vi "Plan Path.vi"(8 "error in (no error)":errorcluster, 10 "Controle":T1, 11 "map reference in":refnum<data-value>) -> (0 "error out":errorcluster, 1 "intensity values":dbl[][](array[numeric]), 2 "Indicator":T1, 3 "map reference out":refnum<data-value>)   [LabVIEW 2012]
uses:
  <vilib>/robotics/Navigation/shared/WorldMap/OccupancyGridWorldMap/NI_Robotics_OccupancyGridWorldMap.lvclass
  <vilib>/robotics/Navigation/NI_Robotics_Navigation .lvlib
panel:
  out "x-y":dbl[][](array[numeric])
  out "goal node":cluster{"X":i32, "Y":i32}={"X"=32, "Y"=32}
  out "start node":cluster{"X":i32, "Y":i32}={"X"=3, "Y"=3}
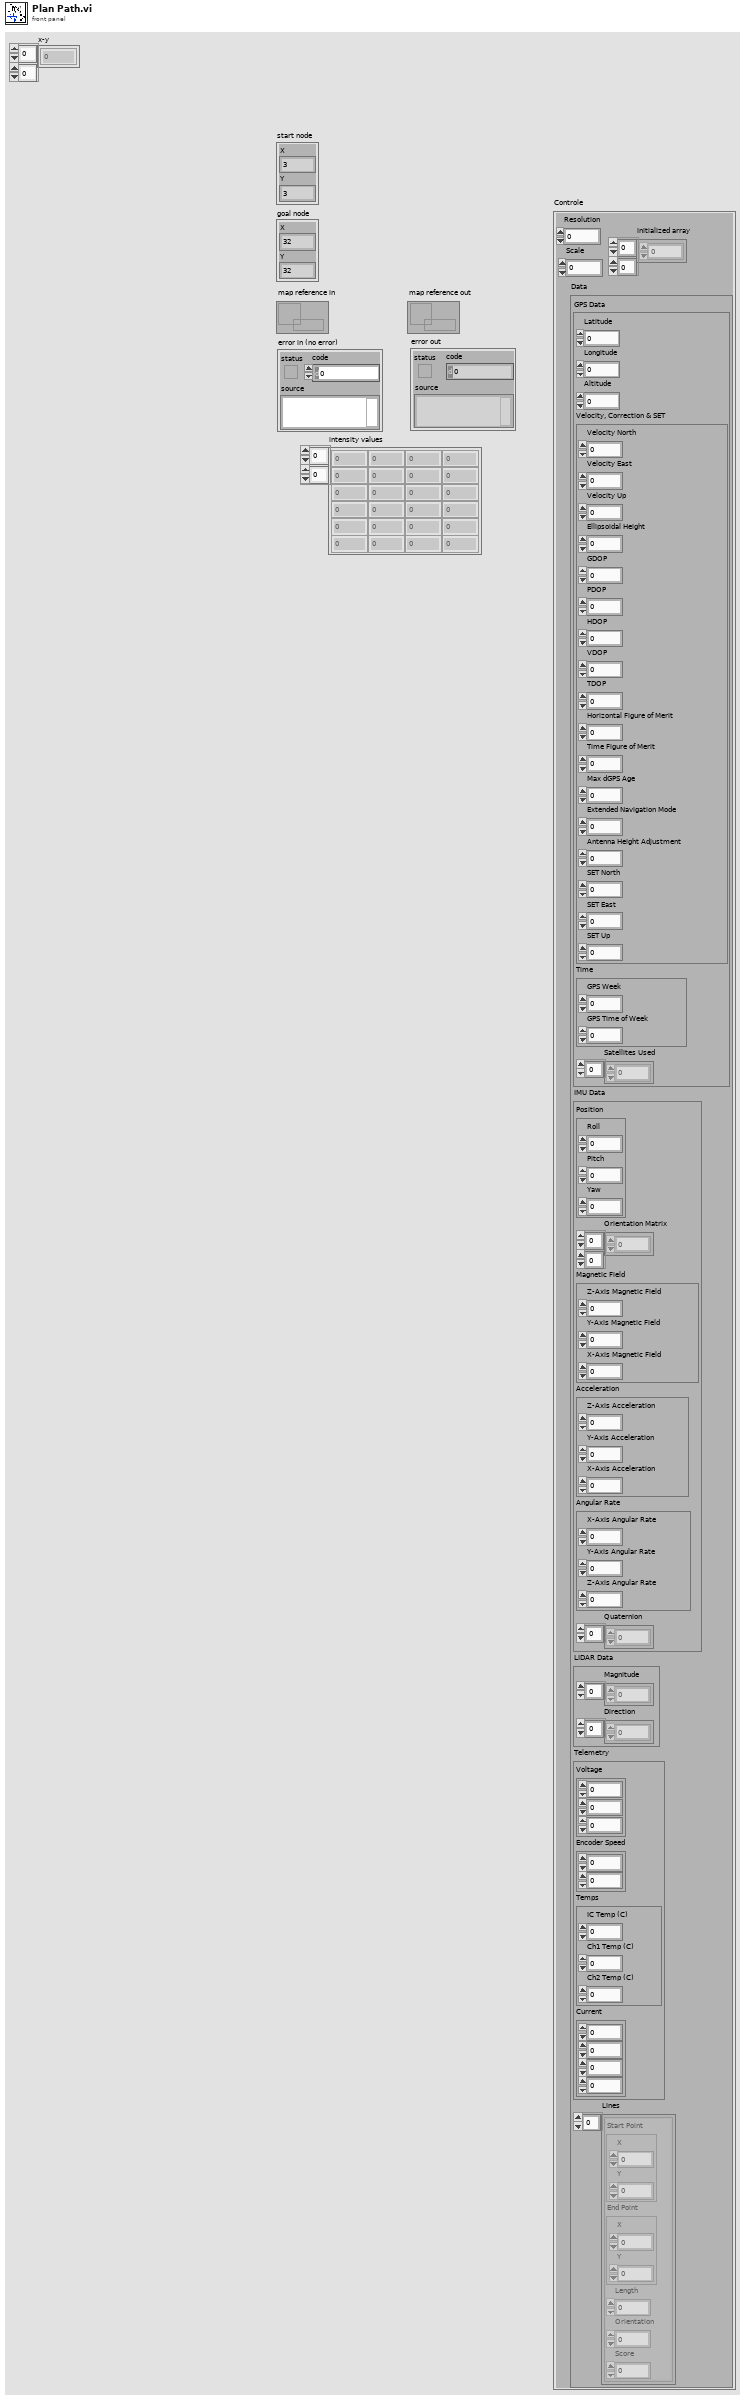
[diagram p1: front panel]
types:
  T1 = cluster{"Resolution":i32, "Scale":dbl, "Data":cluster{"GPS Data":cluster{"Latitude":dbl, "Longitude":dbl, "Altitude":dbl, "Velocity, Correction & SET":cluster{"Velocity North":dbl, "Velocity East":dbl, "Velocity Up":dbl, "Ellipsoidal Height":dbl, "GDOP":sgl, "PDOP":sgl, "HDOP":sgl, "VDOP":sgl, "TDOP":sgl, "Horizontal Figure of Merit":u8, "Time Figure of Merit":u8, "Max dGPS Age":sgl, "Extended Navigation Mode":u8, "Antenna Height Adjustment ":dbl, "SET North":i32, "SET East":i32, "SET Up":i32}, "Time":cluster{"GPS Week":u16, "GPS Time of Week":sgl}, "Satellites Used":i32[]}, "IMU Data":cluster{"Position":cluster{"Roll":dbl, "Pitch":dbl, "Yaw":dbl}, "Orientation Matrix":dbl[][], "Magnetic Field":cluster{"Z-Axis Magnetic Field":dbl, "Y-Axis Magnetic Field":dbl, "X-Axis Magnetic Field":dbl}, "Acceleration":cluster{"Z-Axis Acceleration":dbl, "Y-Axis Acceleration":dbl, "X-Axis Acceleration":dbl}, "Angular Rate":cluster{"X-Axis Angular Rate":dbl, "Y-Axis Angular Rate":dbl, "Z-Axis Angular Rate":dbl}, "Quaternion":dbl[]}, "LIDAR Data":cluster{"Magnitude":dbl[], "Direction":dbl[]}, "Telemetry":cluster{"Voltage":cluster{sgl, sgl, sgl}, "Encoder Speed":cluster{i32, i32}, "Temps":cluster{"IC Temp (C)":i32, "Ch1 Temp (C)":i32, "Ch2 Temp (C)":i32}, "Current":cluster{dbl, dbl, dbl, dbl}}, "Lines":cluster{"Start Point":cluster{"X":sgl, "Y":sgl}, "End Point":cluster{"X":sgl, "Y":sgl}, "Length":dbl, "Orientation":dbl, "Score":dbl}[]}, "initialized array":dbl[][]}
  T2 = cluster{"Latitude":dbl, "Longitude":dbl, "Altitude":dbl, "Velocity, Correction & SET":cluster{"Velocity North":dbl, "Velocity East":dbl, "Velocity Up":dbl, "Ellipsoidal Height":dbl, "GDOP":sgl, "PDOP":sgl, "HDOP":sgl, "VDOP":sgl, "TDOP":sgl, "Horizontal Figure of Merit":u8, "Time Figure of Merit":u8, "Max dGPS Age":sgl, "Extended Navigation Mode":u8, "Antenna Height Adjustment ":dbl, "SET North":i32, "SET East":i32, "SET Up":i32}, "Time":cluster{"GPS Week":u16, "GPS Time of Week":sgl}, "Satellites Used":i32[]}
  T3 = cluster{"Position":cluster{"Roll":dbl, "Pitch":dbl, "Yaw":dbl}, "Orientation Matrix":dbl[][], "Magnetic Field":cluster{"Z-Axis Magnetic Field":dbl, "Y-Axis Magnetic Field":dbl, "X-Axis Magnetic Field":dbl}, "Acceleration":cluster{"Z-Axis Acceleration":dbl, "Y-Axis Acceleration":dbl, "X-Axis Acceleration":dbl}, "Angular Rate":cluster{"X-Axis Angular Rate":dbl, "Y-Axis Angular Rate":dbl, "Z-Axis Angular Rate":dbl}, "Quaternion":dbl[]}
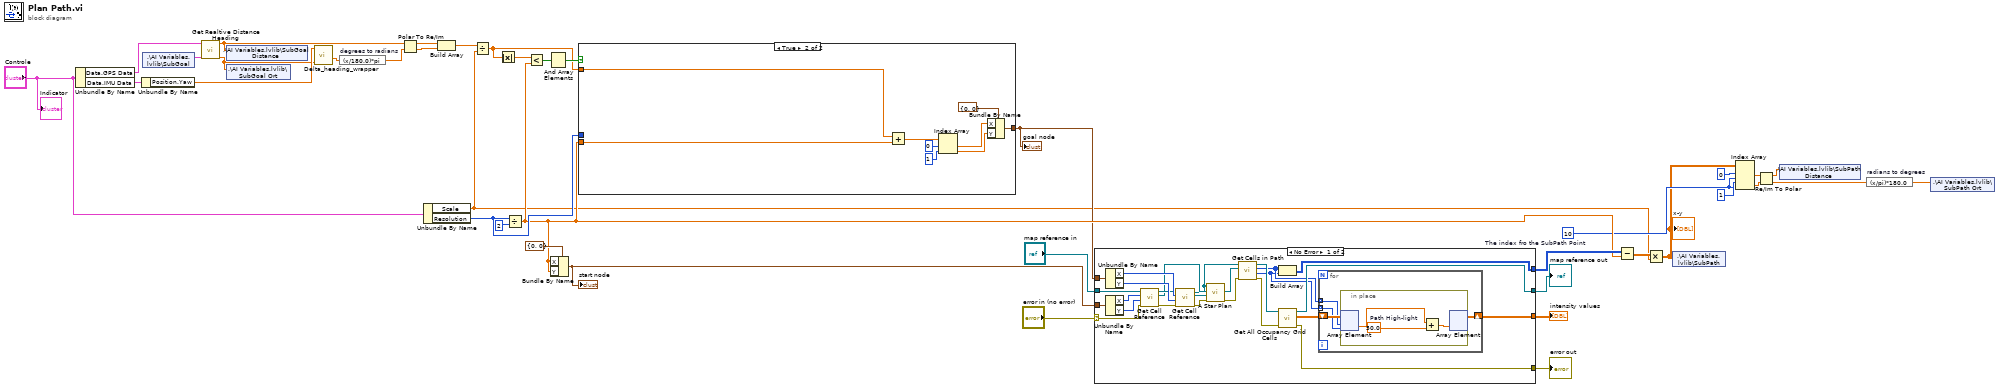
[diagram p0: block diagram]
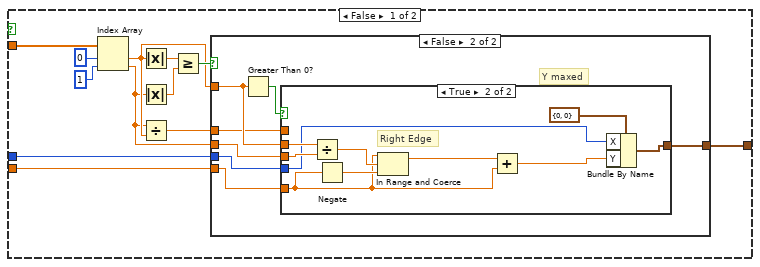
[diagram p2: hidden frame]
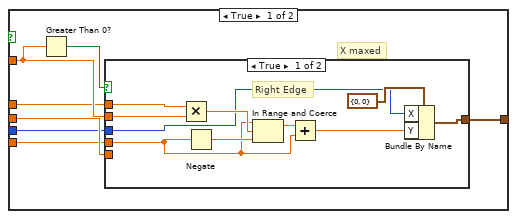
[diagram p3: hidden frame]
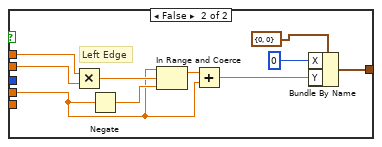
[diagram p4: hidden frame]
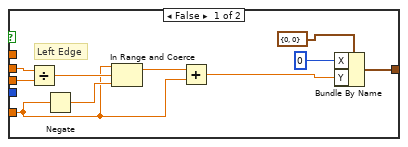
[diagram p5: hidden frame]
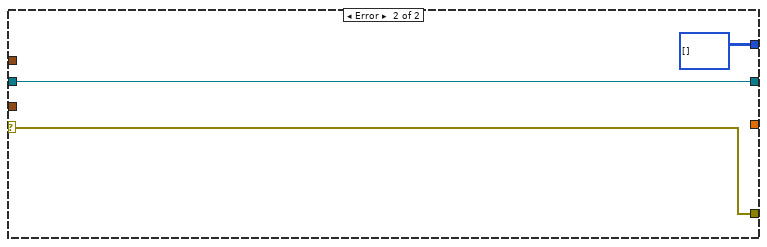
[diagram p6: hidden frame]
diagram:
  w9 = 10  # The index fro the SubPath Point
  n1 = Unbundle By Name("Controle") -> ("Data.GPS Data"=w12:T2, "Data.IMU Data"=w15:T3)
  n2 = Unbundle By Name(w15) -> ("Position.Yaw"=w11:dbl)
  n3 = shared-variable ".\\AI Variables.lvlib\\SubGoal"() -> (w13:T2)  [unwired: 1 in, 1 out]
  n4 = call "Get Realtive Distance Heading.vi"("Goal Position"=w13, "Current Position"=w12) -> ("Bearing"=w1:dbl, "distance (m)"=w5:dbl)  [unwired: 8 in]
  n5 = shared-variable ".\\AI Variables.lvlib\\SubGoal Distance"(w5) -> ()  [unwired: 1 in, 1 out]
  n6 = shared-variable ".\\AI Variables.lvlib\\SubGoal Ort"(w1) -> ()  [unwired: 1 in, 1 out]
  n7 = call "Delta_heading_wrapper.vi"("Goal Heading"=w1, "Robot Heading"=w11) -> ("Heading Adjustment"=w10:dbl)  [unwired: 9 in]
  n8 = expression code="(x/180.0)*pi" "degrees to radians"(w10) -> (w18:dbl)
  n9 = Polar To Re/Im(2:w18, 3:w5) -> (0:w16:dbl, 1:w17:dbl)
  n10 = Unbundle By Name("Controle") -> ("Scale"=w2:dbl, "Resolution"=w22:i32)
  n11 = Build Array(w17, w16) -> (w21:dbl[])
  n12 = Divide(x=w21, y=w2) -> (x/y=w23:dbl[])
  n13 = Absolute Value(x=w23) -> (abs(x)=w24:dbl[])
  n14 = Divide(x=w22, y=2 ("value")) -> (x/y=w20:dbl)
  n15 = Less?(x=w24, y=w20) -> (x < y?=w33:bool[])
  n16 = And Array Elements(Boolean array=w33) -> (logical AND=w34:bool)
  n17 = Bundle By Name(cluster=cluster{"X":i32, "Y":i32} {"X"=0, "Y"=0} ("goal node"), "X"=w20, "Y"=w20) -> (w31:cluster{"X":i32, "Y":i32})
  "start node" <- w31
  n18 = case shown="True" w34 {
    tunnel: w23 -> [w42 w114]
    tunnel: [w43 w107] -> w19
    tunnel: w22 -> [w41 _]
    tunnel: w20 -> [w40 w106]
    frame False {
      n19 = Index Array(array=w42, index #1=0 ("index"), index #2=1 ("index")) -> (element #1=w46:dbl, element #2=w45:dbl)
      n20 = Absolute Value(x=w46) -> (abs(x)=w49:dbl)
      n21 = Absolute Value(x=w45) -> (abs(x)=w48:dbl)
      n22 = Divide(x=w45, y=w46) -> (x/y=w44:dbl)
      n23 = Greater Or Equal?(x=w49, y=w48) -> (x >= y?=w47:bool)
      n24 = case shown="False" w47 {
        tunnel: w46 -> [w56 w83]
        tunnel: w45 -> [w55 w82]
        tunnel: w44 -> [w54 w81]
        tunnel: [w57 w84] -> w43
        tunnel: w41 -> [w53 w80]
        tunnel: w40 -> [w52 w79]
        frame True {
          # "X maxed"
          n25 = Greater Than 0?(x=w56) -> (x > 0?=w58:bool)
          n26 = case shown="True" w58 {
            tunnel: [w67 w77] -> w57
            tunnel: w56 -> [w65 w75]
            tunnel: w55 -> [_ _]
            tunnel: w54 -> [w66 w76]
            tunnel: w53 -> [w62 _]
            tunnel: w52 -> [w59 w70]
            frame True {
              # "Right Edge"
              n27 = Multiply(x=w66, y=w65) -> (x*y=w64:dbl)
              n28 = Negate(x=w59) -> (-x=w60:dbl)
              n29 = In Range and Coerce(upper limit=w59, x=w64, lower limit=w60) -> (coerced(x)=w63:dbl)  [unwired: 1 out]
              n30 = Add(x=w63, y=w59) -> (x+y=w61:dbl)
              n31 = Bundle By Name(cluster=cluster{"X":i32, "Y":i32} {"X"=0, "Y"=0} ("goal node"), "X"=w62, "Y"=w61) -> (w67:cluster{"X":i32, "Y":i32})
            }
            frame False {
              # "Left Edge"
              n32 = Multiply(x=w76, y=w75) -> (x*y=w74:dbl)
              n33 = Negate(x=w70) -> (-x=w71:dbl)
              n34 = In Range and Coerce(upper limit=w70, x=w74, lower limit=w71) -> (coerced(x)=w73:dbl)  [unwired: 1 out]
              n35 = Add(x=w73, y=w70) -> (x+y=w72:dbl)
              n36 = Bundle By Name(cluster=cluster{"X":i32, "Y":i32} {"X"=0, "Y"=0} ("goal node"), "X"=0, "Y"=w72) -> (w77:cluster{"X":i32, "Y":i32})
            }
          }
        }
        frame False {
          # "Y maxed"
          n37 = Greater Than 0?(x=w83) -> (x > 0?=w85:bool)
          n38 = case shown="True" w85 {
            tunnel: [w94 w104] -> w84
            tunnel: w83 -> [w87 w98]
            tunnel: w82 -> [w86 w97]
            tunnel: w81 -> [_ _]
            tunnel: w80 -> [_ w96]
            tunnel: w79 -> [w89 w99]
            frame False {
              # "Left Edge"
              n39 = Divide(x=w87, y=w86) -> (x/y=w93:dbl)
              n40 = Negate(x=w89) -> (-x=w90:dbl)
              n41 = In Range and Coerce(upper limit=w89, x=w93, lower limit=w90) -> (coerced(x)=w92:dbl)  [unwired: 1 out]
              n42 = Add(x=w92, y=w89) -> (x+y=w91:dbl)
              n43 = Bundle By Name(cluster=cluster{"X":i32, "Y":i32} {"X"=0, "Y"=0} ("goal node"), "X"=0, "Y"=w91) -> (w94:cluster{"X":i32, "Y":i32})
            }
            frame True {
              # "Right Edge"
              n44 = Divide(x=w98, y=w97) -> (x/y=w103:dbl)
              n45 = Negate(x=w99) -> (-x=w100:dbl)
              n46 = In Range and Coerce(upper limit=w99, x=w103, lower limit=w100) -> (coerced(x)=w102:dbl)  [unwired: 1 out]
              n47 = Add(x=w102, y=w99) -> (x+y=w101:dbl)
              n48 = Bundle By Name(cluster=cluster{"X":i32, "Y":i32} {"X"=0, "Y"=0} ("goal node"), "X"=w96, "Y"=w101) -> (w104:cluster{"X":i32, "Y":i32})
            }
          }
        }
      }
    }
    frame True {
      n49 = Add(x=w114, y=w106) -> (x+y=w112:dbl[])
      n50 = Index Array(array=w112, index #1=0 ("index"), index #2=1 ("index")) -> (element #1=w109:dbl, element #2=w108:dbl)
      n51 = Bundle By Name(cluster=cluster{"X":i32, "Y":i32} {"X"=0, "Y"=0} ("goal node"), "X"=w109, "Y"=w108) -> (w107:cluster{"X":i32, "Y":i32})
    }
  }
  "goal node" <- w19
  n52 = case shown="No Error" "error in (no error)" {
    selector: "error in (no error)" -> [w124 w148]
    tunnel: "map reference in" -> [w125 w149]
    tunnel: w19 -> [w123 _]
    tunnel: w31 -> [w122 _]
    tunnel: [w121 _] -> w39
    tunnel: [w120 w149] -> w37
    tunnel: [w119 w148] -> w36
    tunnel: [w116 i32[][] []] -> w25
    frame No Error {
      n53 = Unbundle By Name(w123) -> ("X"=w138:i32, "Y"=w139:i32)
      n54 = Unbundle By Name(w122) -> ("X"=w136:i32, "Y"=w137:i32)
      n55 = call <vilib>:"Get Cell Reference.vi"("error in (no error)"=w124, "y"=w137, "x"=w136, "map reference in"=w125) -> ("error out"=w129:errorcluster, "cell reference"=w127:refnum<data-value>, "map reference out"=w132:refnum<data-value>)  [unwired: 4 in, 1 out]
      n56 = call <vilib>:"Get Cell Reference.vi"("error in (no error)"=w129, "y"=w139, "x"=w138, "map reference in"=w132) -> ("error out"=w133:errorcluster, "cell reference"=w126:refnum<data-value>, "map reference out"=w115:refnum<data-value>)  [unwired: 4 in, 1 out]
      n57 = call <vilib>:"A Star Plan.vi"("error in (no error)"=w133, "goal reference"=w126, "start reference"=w127, "map reference in"=w115) -> ("error out"=w134:errorcluster, "path references"=w131:refnum<data-value>[])  [unwired: 4 in, 2 out]
      n58 = call <vilib>:"Get Cells in Path.vi"("error in (no error)"=w134, "path references"=w131, "map reference in"=w115) -> ("error out"=w128:errorcluster, "y coordinates"=w117:i32[], "x coordinates"=w118:i32[], "map reference out"=w130:refnum<data-value>)  [unwired: 5 in]
      n59 = Build Array(w118, w117) -> (w116:i32[][])
      n60 = call <vilib>:"Get All Occupancy Grid Cells.vi"("error in (no error)"=w128, "map reference in"=w130) -> ("error out"=w119:errorcluster, "occupancy grid"=w135:dbl[][], "map reference out"=w120:refnum<data-value>)  [unwired: 7 in]
      n61 = for {
        tunnel: w117 -> [w141] mode=indexing
        tunnel: w118 -> [w142] mode=indexing
        shift-right: [w140] -> w121
        shift-left: w135 -> [w143]
        n62 = in-place {
          w146 = 50.0  # Path High-light
          n63 = in-place-array #1(w143, w142, w141) -> (w145:dbl)
          n64 = Add(x=w145, y=w146) -> (x+y=w144:dbl)
          n65 = in-place-array #1(w144) -> (w140:dbl[][])  [unwired: 2 out]
        }
      }
    }
    frame Error {
    }
  }
  "map reference out" <- w37
  "error out" <- w36
  "intensity values" <- w39
  n66 = Subtract(x=w25, y=w20) -> (x-y=w3:dbl[][])
  n67 = Multiply(x=w3, y=w2) -> (x*y=w4:dbl[][])
  "x-y" <- w4
  n68 = shared-variable ".\\AI Variables.lvlib\\SubPath"(w4) -> ()  [unwired: 1 in, 1 out]
  n69 = Index Array(array=w4, index (row) #1=0 ("index (row)"), index (col) #1=w9, index (row) #2=1 ("index (row)"), index (col) #2=w9) -> (element #1=w27:dbl, element #2=w26:dbl)
  n70 = Re/Im To Polar(2:w26, 3:w27) -> (0:w7:dbl, 1:w8:dbl)
  n71 = shared-variable ".\\AI Variables.lvlib\\SubPath Distance"(w8) -> ()  [unwired: 1 in, 1 out]
  n72 = expression code="(x/pi)*180.0" "radians to degrees"(w7) -> (w6:dbl)
  n73 = shared-variable ".\\AI Variables.lvlib\\SubPath Ort"(w6) -> ()  [unwired: 1 in, 1 out]
  "Indicator" <- "Controle"
